vi "get screen size.vi"(4 "screen":i32) -> (0 "wind size (width/height)":T1, 1 "height":i16, 2 "width":i16)   [LabVIEW 2011]
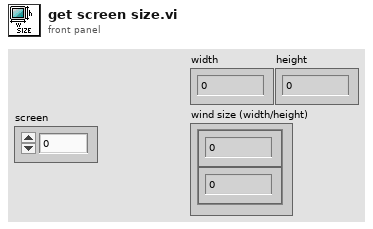
[diagram p1: front panel]
types:
  T1 = cluster{"Numeric Control":i16, "Numeric Control":i16}
  T2 = typedef "LVAllMonitorsDisplayTypeDef.ctl" = cluster{"Bounds":cluster{"Left":i16, "Top":i16, "Right":i16, "Bottom":i16}, "Depth":i16}[]
  T3 = cluster{"Bounds":cluster{"Left":i16, "Top":i16, "Right":i16, "Bottom":i16}, "Depth":i16}
  T4 = cluster{"Left":i16, "Top":i16, "Right":i16, "Bottom":i16}
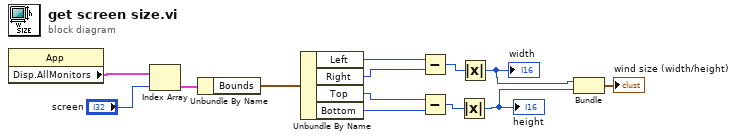
[diagram p0: block diagram]
diagram:
  n1 = property class="App"() -> ("Disp.AllMonitors"=w13:T2)  [unwired: 2 in, 2 out]
  n2 = Index Array(array=w13, index="screen") -> (element=w5:T3)
  n3 = Unbundle By Name(w5) -> ("Bounds"=w12:T4)
  n4 = Unbundle By Name(w12) -> ("Left"=w11:i16, "Right"=w8:i16, "Top"=w7:i16, "Bottom"=w6:i16)
  n5 = Subtract(x=w11, y=w8) -> (x-y=w10:i16)
  n6 = Subtract(x=w7, y=w6) -> (x-y=w9:i16)
  n7 = Absolute Value(x=w9) -> (abs(x)=w2:i16)
  "height" <- w2
  n8 = Absolute Value(x=w10) -> (abs(x)=w3:i16)
  "width" <- w3
  n9 = Bundle(w3, w2) -> (→"wind size (width/height)":cluster{i16, i16})  [unwired: 1 in]
